vi "capacitance navigation v2.1.vi"() -> ()   [LabVIEW 2021]
uses:
  <userlib>/Nanonis Prog Interface V5/Nanonis Prog Interface.lvlib
panel:
  out "Delta reached?":bool
  out "Cap reached?":bool
  in  "Cap threshold (pA)":dbl
  in  "Delta cap threshold (pA)":dbl
  in  "pause":bool
  in  "Delete First Entry":bool
  in  "Time between averages (ms)":u32
  out "Avg index":i32
  in  "Averages":i32=50
  in  "milliseconds to wait":u32=1000
  in  "stop":bool
  in  "?":bool
  in  "Max Steps":u16=500
  in  "Direction":enum16{"X +", "X -", "Y +", "Y -", "Z +", "Z -"}(ring)
  out "Delta":cluster{"index":i32, sgl}[](graph)
  in  "Number of Steps":u16=50
  out "Capacitance":cluster{"index":i32, sgl}[](graph)
  in  "Frequency (Hz)":sgl=261.0
  in  "Amplitude (V)":sgl=260.0
  # "Threshold only works \nin Z+ direction"
  # "Max Steps On"
  # "Max Steps Off"
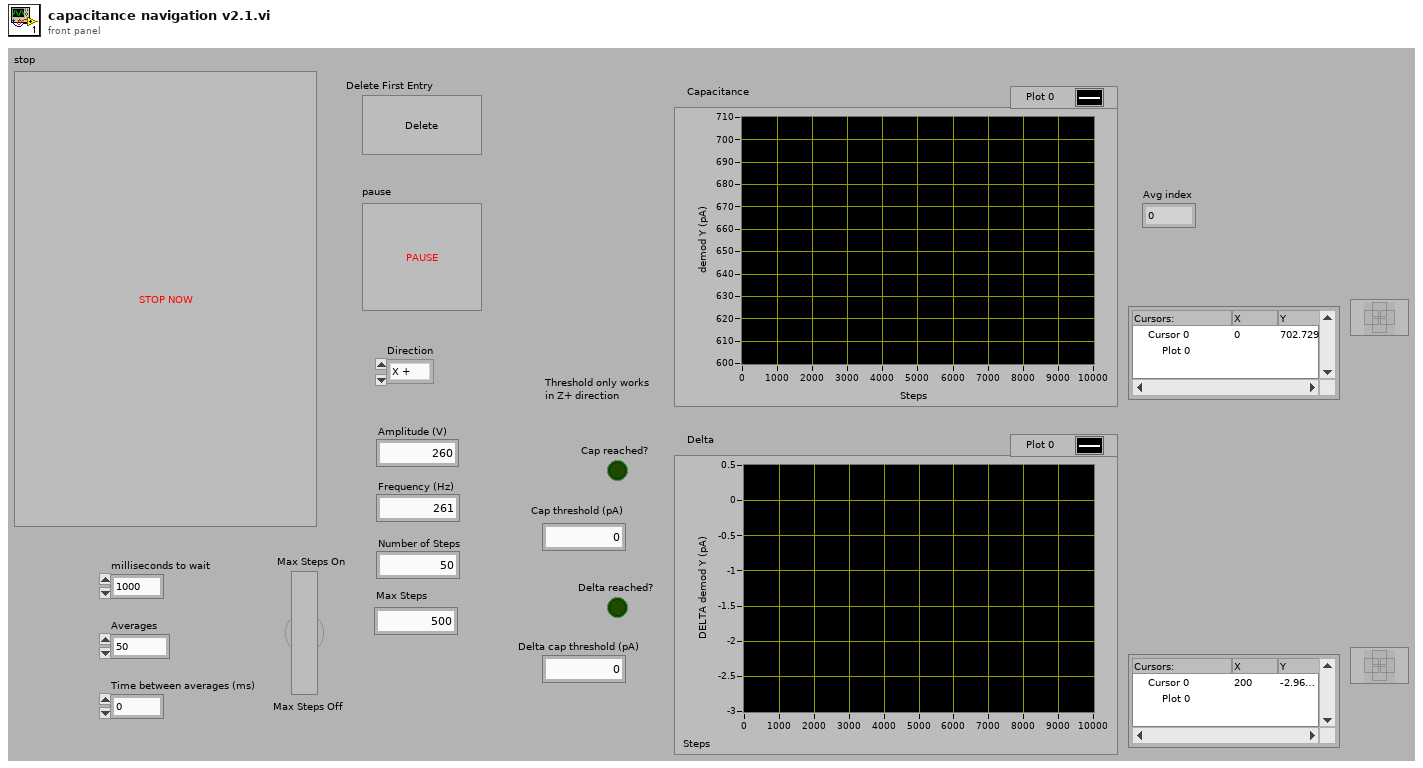
[diagram p1: front panel]
types:
  T1 = enum8{"Group 1", "Group 2", "Group 3", "Group 4", "Group 5", "Group 6"}
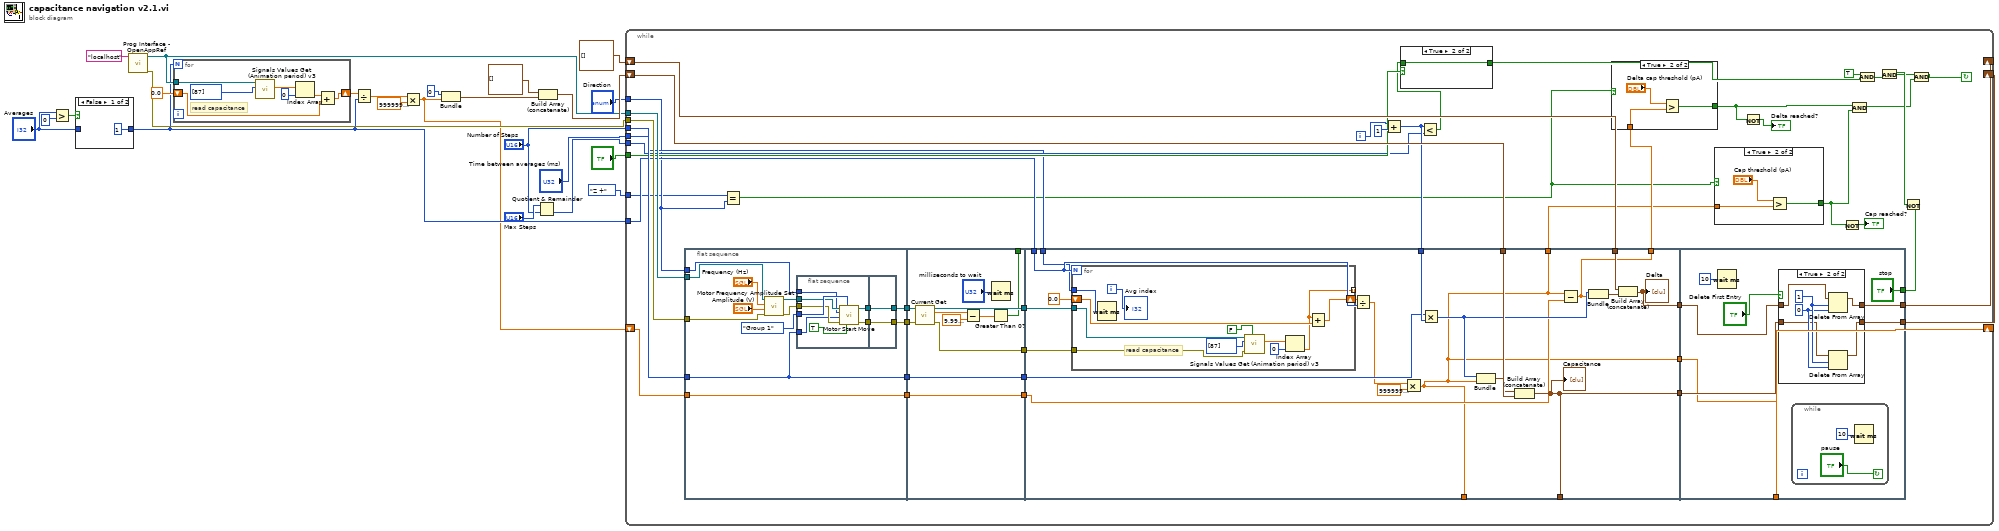
[diagram p0: block diagram]
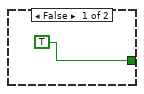
[diagram p3: hidden frame]
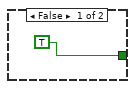
[diagram p4: hidden frame]
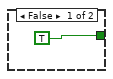
[diagram p5: hidden frame]
diagram:
  n1 = Greater?(x="Averages", y=0) -> (0:w9:bool)
  n2 = case shown="False" w9 {
    tunnel: "Averages" -> [_ w26]
    tunnel: [1 ("Averages") w26] -> w4
    frame False {
    }
    frame True {
    }
  }
  n3 = call <userlib>:"Prog Interface - OpenAppRef.vi"("Machine name (local machine IP)"="localhost" ("machine name (localhost)")) -> ("Error out"=w18:errorcluster, "Application reference"=w17:refnum<vi>)  [unwired: 5 in]
  n4 = for {
    N: w4 -> [_]
    tunnel: w17 -> [w30]
    shift-right: [w27] -> w5
    shift-left: sgl 0.0 ("Internal Ch Value") -> [w29]
    # "read capacitance"
    n5 = call <userlib>:"Signals Values Get (Animation period) v3.vi"("Signals indexes (0-127)"=i8[] [87], "Application ref in"=w30) -> ("Signals Values"=w31:sgl[])  [unwired: 6 in, 2 out]
    n6 = Index Array(array=w31, index=0) -> (element=w28:sgl)
    n7 = Add(x=w28, y=w29) -> (x+y=w27:sgl)
  }
  n8 = Divide(x=w5, y=w4) -> (x/y=w3:sgl)
  n9 = Multiply(x=w3, y=sgl 1000000000000.0) -> (x*y=w2:sgl)
  n10 = Bundle("index"=0, w2) -> (w21:cluster{"index":i32, sgl})  [unwired: 1 in]
  n11 = Quotient & Remainder(x="Max Steps", y="Number of Steps") -> (floor(x/y)=w12:u16)  [unwired: 1 out]
  n12 = Build Array (concatenate)(cluster{i32, sgl}[] [], w21) -> (w20:cluster{"index":i32, sgl}[])
  n13 = while {
    shift-right: [w50] -> _
    shift-left: w20 -> [w76]
    tunnel: w17 -> [w74]
    tunnel: w18 -> [w73]
    shift-right: [w67] -> _
    shift-left: cluster{i32, sgl}[] [] -> [w66]
    tunnel: "Direction" -> [w36]
    tunnel: "Number of Steps" -> [w65]
    tunnel: w12 -> [w58]
    tunnel: "?" -> [w64]
    tunnel: w4 -> [w53]
    tunnel: "Time between averages (ms)" -> [w52]
    shift-right: [w48] -> _
    shift-left: w2 -> [w47]
    tunnel: enum16{"X +", "X -", "Y +", "Y -", "Z +", "Z -"}."Z +" ("Direction") -> [w35]
    i -> [w61]
    stop <- w43 continue-if-true
    n14 = flat-sequence {
      tunnel: [w91] -> w78
      tunnel: w74 -> [w94]
      tunnel: w73 -> [w97]
      tunnel: [w96] -> w72
      tunnel: [w95] -> w71
      tunnel: w36 -> [w90]
      tunnel: w65 -> [w91]
      tunnel: w47 -> [w89]
      tunnel: [w89] -> w46
      tunnel: w78 -> [w123]
      tunnel: [w123] -> w77
      tunnel: w72 -> [w122]
      tunnel: w71 -> [w121]
      tunnel: [w120] -> w70
      tunnel: [w119] -> w69
      tunnel: [w116] -> _
      tunnel: w46 -> [w113]
      tunnel: [w113] -> w45
      tunnel: [w127] -> _
      tunnel: w59 -> [w142]
      tunnel: w77 -> [w139]
      tunnel: w76 -> [w140]
      tunnel: [w124] -> _
      tunnel: w70 -> [w138]
      tunnel: w69 -> [w137]
      tunnel: [w133] -> w68
      tunnel: w66 -> [w134]
      tunnel: w53 -> [w129]
      tunnel: w52 -> [w128]
      tunnel: [w127] -> w51
      tunnel: [w124] -> w49
      tunnel: w45 -> [w126]
      tunnel: [w125] -> w44
      tunnel: [w124] -> w42
      tunnel: w68 -> [w160]
      tunnel: [w159] -> w67
      tunnel: ["stop"] -> w54
      tunnel: [w157] -> w50
      tunnel: w51 -> [w158]
      tunnel: w49 -> [w156]
      tunnel: [w156] -> w48
      frame #0 {
        n15 = call <userlib>:"Motor Frequency Amplitude Set.vi"("Error in (no error)"=w97, "Amplitude (V) (NaN=no change)"="Amplitude (V)", "Frequency (Hz) (NaN=no change)"="Frequency (Hz)", "Application ref in"=w94) -> ("Error out"=w98:errorcluster, "Application ref out"=w99:refnum<vi>)  [unwired: 6 in]
        n16 = flat-sequence {
          tunnel: T1."Group 1" ("Group") -> [w109]
          tunnel: w99 -> [w108]
          tunnel: w98 -> [w107]
          tunnel: w91 -> [w106]
          tunnel: [w105] -> w93
          tunnel: [w104] -> w92
          tunnel: w90 -> [w103]
          tunnel: [w111] -> w95
          tunnel: [w112] -> w96
          tunnel: w93 -> [w112]
          tunnel: w92 -> [w111]
          frame #0 {
            n17 = call <userlib>:"Motor Start Move.vi"("Wait until finished? (F)"=TRUE, "Group"=w109, "Error in (no error)"=w107, "Number of steps"=w106, "Direction"=w103, "Application ref in"=w108) -> ("Error out"=w104:errorcluster, "Application ref out"=w105:refnum<vi>)  [unwired: 3 in]
          }
          frame #1 {
          }
        }
      }
      frame #1 {
        n18 = call <userlib>:"Current Get.vi"("Error in (no error)"=w121, "Application ref in"=w122) -> ("Error out"=w120:errorcluster, "Current (A)"=w118:sgl, "Application ref out"=w119:refnum<vi>)  [unwired: 5 in]
        n19 = Subtract(x=w118, y=sgl 1e-09) -> (x-y=w117:sgl)
        n20 = Greater Than 0?(x=w117) -> (x > 0?=w116:bool)
        n21 = Wait (ms)(milliseconds to wait="milliseconds to wait") -> ()  [unwired: 1 out]
      }
      frame #2 {
        n22 = for {
          N: w129 -> [_]
          tunnel: w138 -> [w151]
          tunnel: w137 -> [w150]
          shift-right: [w148] -> w131
          shift-left: sgl 0.0 ("y") -> [w149]
          tunnel: w128 -> [w146]
          tunnel: [w144] -> _ mode=indexing
          i -> [w147]
          # "read capacitance"
          n23 = Wait (ms)(milliseconds to wait=w146) -> ()  [unwired: 1 out]
          n24 = call <userlib>:"Signals Values Get (Animation period) v3.vi"("Wait for newest data (F=False)"=FALSE, "error in (no error)"=w151, "Signals indexes (0-127)"=i8[] [87], "Application ref in"=w150) -> ("Signals Values"=w152:sgl[])  [unwired: 4 in, 2 out]
          n25 = Index Array(array=w152, index=0) -> (element=w144:sgl)
          n26 = Add(x=w144, y=w149) -> (x+y=w148:sgl)
          "Avg index" <- w147
        }
        n27 = Divide(x=w131, y=w129) -> (x/y=w130:sgl)
        n28 = Multiply(x=w130, y=sgl 1000000000000.0) -> (x*y=w124:sgl)
        n29 = Multiply(x=w139, y=w142) -> (x*y=w136:i32)
        n30 = Bundle(w136, w124) -> (w141:cluster{i32, sgl})  [unwired: 1 in]
        n31 = Build Array (concatenate)(w140, w141) -> (w127:cluster{"index":i32, sgl}[])
        "Capacitance" <- w127
        n32 = Subtract(x=w124, y=w126) -> (x-y=w125:sgl)
        n33 = Bundle(w136, w125) -> (w135:cluster{i32, sgl})  [unwired: 1 in]
        n34 = Build Array (concatenate)(w134, w135) -> (w133:cluster{i32, sgl}[])
        "Delta" <- w133
      }
      frame #3 {
        n35 = Wait (ms)(milliseconds to wait=u32 10) -> ()  [unwired: 1 out]
        n36 = case shown="True" "Delete First Entry" {
          tunnel: w160 -> [w166 w170]
          tunnel: [w166 w169] -> w159
          tunnel: w158 -> [w165 w167]
          tunnel: [w165 w168] -> w157
          frame False {
          }
          frame True {
            w172 = 1 ("length")
            w171 = 0 ("index")
            n37 = Delete From Array(array=w170, length=w172, index=w171) -> (array with subset deleted=w169:cluster{i32, sgl}[])  [unwired: 1 out]
            n38 = Delete From Array(array=w167, length=w172, index=w171) -> (array with subset deleted=w168:cluster{"index":i32, sgl}[])  [unwired: 1 out]
          }
        }
        n39 = while {
          stop <- "pause" continue-if-true
          n40 = Wait (ms)(milliseconds to wait=u32 10) -> ()  [unwired: 1 out]
        }
      }
    }
    n41 = Equal?(x=w35, y=w36) -> (x = y?=w34:bool)
    n42 = Add(x=w61, y=u16 1) -> (x+y=w59:i32)
    n43 = Less?(x=w59, y=w58) -> (x < y?=w60:bool)
    n44 = case shown="True" w64 {
      tunnel: w60 -> [_ w88]
      tunnel: [TRUE w88] -> w62
      frame False {
      }
      frame True {
      }
    }
    n45 = case shown="True" w34 {
      tunnel: w44 -> [_ w86]
      tunnel: [TRUE w84] -> w40
      frame False {
      }
      frame True {
        n46 = Greater?(x="Delta cap threshold (pA)", y=w86) -> (0:w84:bool)
      }
    }
    n47 = case shown="True" w34 {
      tunnel: w42 -> [_ w81]
      tunnel: [TRUE w80] -> w38
      frame False {
      }
      frame True {
        n48 = Greater?(x="Cap threshold (pA)", y=w81) -> (0:w80:bool)
      }
    }
    n49 = Not(x=w40) -> (.not. x?=→"Delta reached?":bool)
    n50 = Not(x=w38) -> (.not. x?=→"Cap reached?":bool)
    n51 = And(x=w40, y=w38) -> (x .and. y?=w41:bool)
    n52 = And(x=TRUE, y=w62) -> (x .and. y?=w56:bool)
    n53 = Not(x=w54) -> (.not. x?=w57:bool)
    n54 = And(x=w57, y=w56) -> (x .and. y?=w55:bool)
    n55 = And(x=w55, y=w41) -> (x .and. y?=w43:bool)
  }
